vi "Update M.vi"(8 "error in (no error)":errorcluster, 10 "Update M":string, 11 "Actor M in":refnum<class "Actor M.lvclass">) -> (0 "error out":errorcluster, 3 "Actor M out":refnum<class "Actor M.lvclass">)   [LabVIEW 2019, in "Actor M.lvlib" / "Actor M.lvclass"]
uses:
  Actor M.lvclass
  Actor M.lvclass/Actor M.ctl
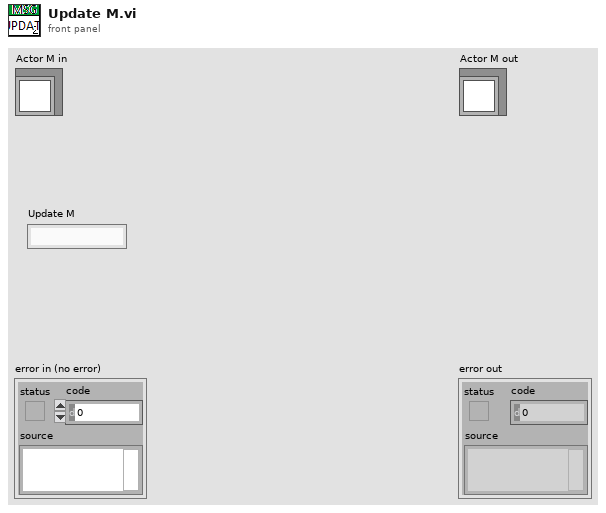
[diagram p1: front panel]
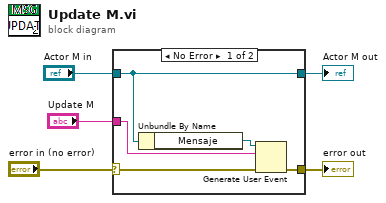
[diagram p0: block diagram]
diagram:
  n1 = case shown="No Error" "error in (no error)" {
    selector: "error in (no error)" -> [w7 w12]
    tunnel: [w6 w12] -> w4
    tunnel: [w10 w11] -> w2
    tunnel: "Actor M in" -> [w10 w11]
    tunnel: "Update M" -> [w8 _]
    frame No Error {
      n2 = Unbundle By Name(w10) -> ("Mensaje"=w9:refnum<user-event>)
      n3 = Generate User Event(user event=w9, event data cluster=w8, error in=w7) -> (error out=w6:errorcluster)  [unwired: 1 in, 1 out]
    }
    frame Error {
    }
  }
  "error out" <- w4
  "Actor M out" <- w2
